vi "fir2_test.vi"() -> ()   [LabVIEW 2013]
uses:
  <vilib>/rvi/FXPMathLib/FxpConvert/subVIs/nifxpmath_Convert_SimConfig.ctl
  <vilib>/fxp/LVFixedPointQuantizationPolicyTypeDef.ctl
  <vilib>/fxp/LVFixedPointOverflowPolicyTypeDef.ctl
  <vilib>/rvi/FXPMathLib/FxpConvert/simVIs/DllFxpConvertTemp_sub.vi
  <vilib>/rvi/FXPMathLib/FxpInterpret/XNode/nifxpmath_Interpret.xnode
  <vilib>/rvi/FXPMathLib/FxpConvert/XNode/nifxpmath_Convert.xnode
panel:
  out "Array 2":fxp<+/-,16,16>[](array[numeric])
  out "logical OR":bool
  out "Array":bool[](array[boolean])
  out "I out":fxp<+/-,16,16>[](array[numeric])
  out "Q out":fxp<+/-,16,16>[](array[numeric])
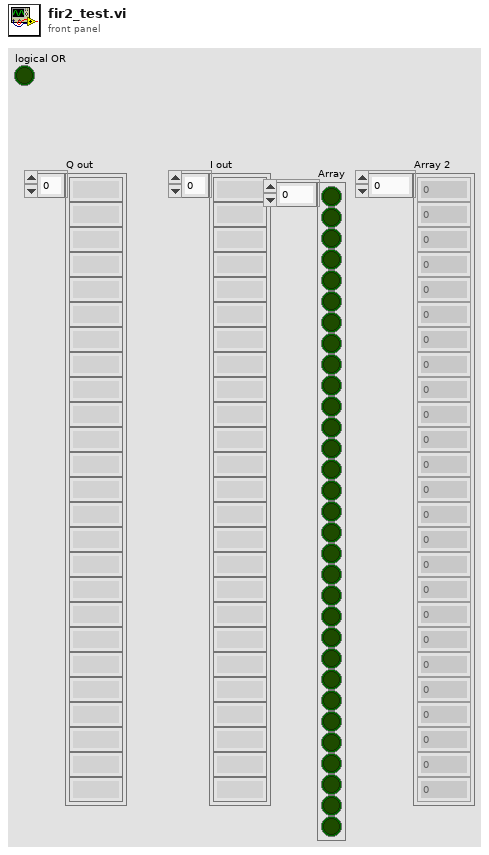
[diagram p1: front panel]
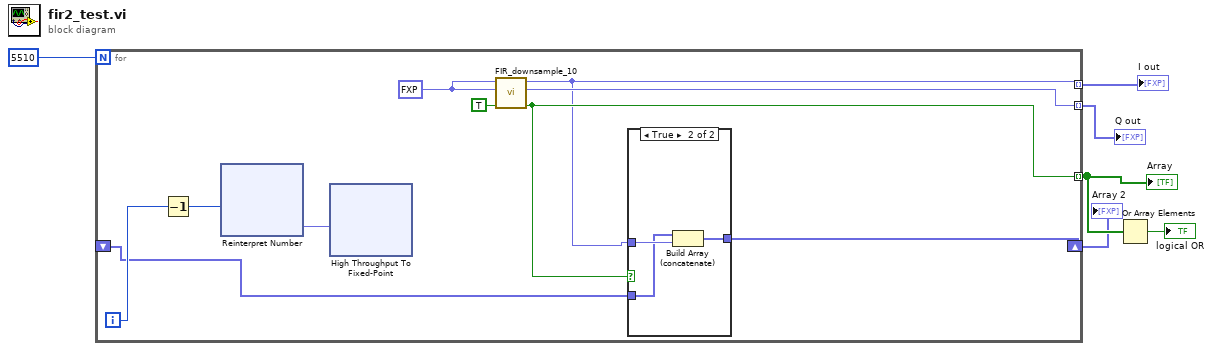
[diagram p0: block diagram]
diagram:
  n1 = for {
    N: 5510 -> [_]
    tunnel: [w7] -> w6 mode=indexing
    tunnel: [w8] -> w5 mode=indexing
    tunnel: [w12] -> w3 mode=indexing
    shift-right: [w11] -> w1
    shift-left: _ -> [w10]
    i -> [w16]
    w9 = fxp<+/-,25,19> 100.0 ("I in")
    n2 = Decrement(x=w16) -> (x-1=w14:i32)
    n3 = xnode "Reinterpret Number"("x"=w14) -> ("y"=w15:fxp<+/-,32,32>)
    n4 = xnode "High Throughput To Fixed-Point"("x"=w15) -> ()  [unwired: 1 out]
    n5 = call "FIR_downsample_10.vi"("valid in"=TRUE, "Q in"=w9, "I in"=w9) -> ("valid out"=w12:bool, "Q out"=w8:fxp<+/-,16,16>, "I out"=w7:fxp<+/-,16,16>)  [unwired: 6 in]
    n6 = case shown="True" w12 {
      tunnel: w7 -> [_ w20]
      tunnel: [w17 w19] -> w11
      tunnel: w10 -> [w17 w18]
      frame False {
      }
      frame True {
        n7 = Build Array (concatenate)(w18, w20) -> (w19:fxp<+/-,16,16>[])
      }
    }
  }
  "Q out" <- w5
  "I out" <- w6
  "Array" <- w3
  "Array 2" <- w1
  n8 = Or Array Elements(Boolean array=w3) -> (logical OR=→"logical OR":bool)
